vi "Main_XXA.vi"() -> ()   [LabVIEW 2024]
uses:
  Utility/Universal Utility/TypeDefs_Utility/Cluster_Row-Column.ctl
panel:
  in  "Use Puzzle":bool
  out "Answer":u32
  in  "Puzzle":string
  in  "Example":string
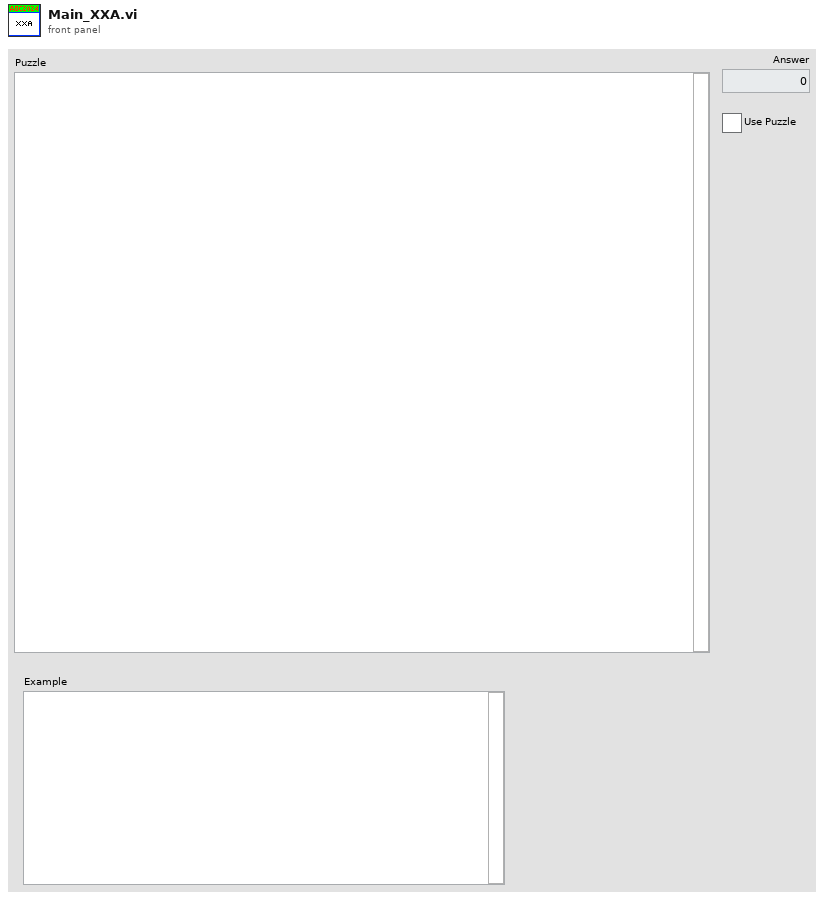
[diagram p1: front panel]
types:
  T1 = typedef "Cluster_Row-Column.ctl" = cluster{"R":i32, "C":i32}
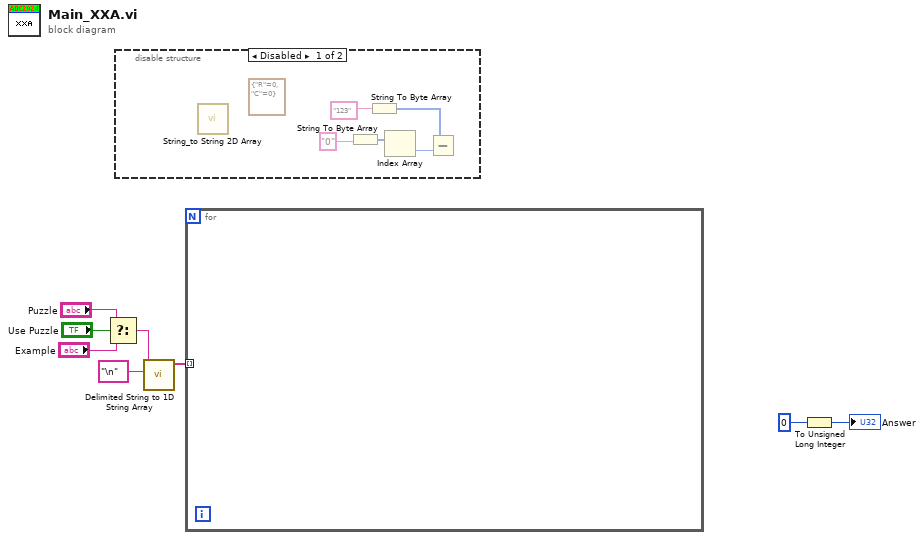
[diagram p0: block diagram]
diagram:
  n1 = Select(t="Puzzle", s="Use Puzzle", f="Example") -> (s? t:f=w4:string)
  n2 = disable-structure shown="Disabled" {
    frame Disabled {
      (unwired) T1 {"R"=0, "C"=0} ("Position")
      n3 = call "String_to String 2D Array.vi"() -> ()  [unwired: 11 in, 1 out]
      n4 = String To Byte Array(string="0") -> (unsigned byte array=w11:u8[])
      n5 = String To Byte Array(string="123") -> (unsigned byte array=w9:u8[])
      n6 = Index Array(array=w11) -> (element=w10:u8)  [unwired: 1 in]
      n7 = Subtract(x=w9, y=w10) -> ()  [unwired: 1 out]
    }
    frame Enabled {
    }
  }
  n8 = call <vilib>:"Delimited String to 1D String Array.vi"("delimiter"="\n" ("delimiter (Tab)"), "delimited string"=w4) -> ("string array"=w7:string[])  [unwired: 9 in]
  n9 = for {
    tunnel: w7 -> [_] mode=indexing
  }
  n10 = To Unsigned Long Integer(number=u32 0) -> (unsigned 32bit integer=→"Answer":u32)
